vi "Bind Port.vi"(6 "timeout ms":i32=1000, 8 "error in":errorcluster, 10 "port":u16, 11 "NetStream in":refnum<class "NetStream.lvclass">) -> (0 "error out":errorcluster, 2 "Remote connected?":bool, 3 "NetStream out":refnum<class "NetStream.lvclass">)   [LabVIEW 2014, in "hse-network.lvlib" / "NetStream.lvclass"]
uses:
  NetStream.lvclass
  NetStream.lvclass/NetStream.ctl
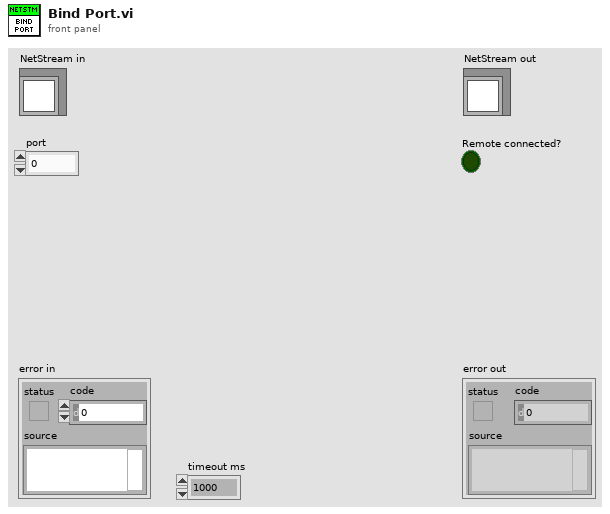
[diagram p1: front panel]
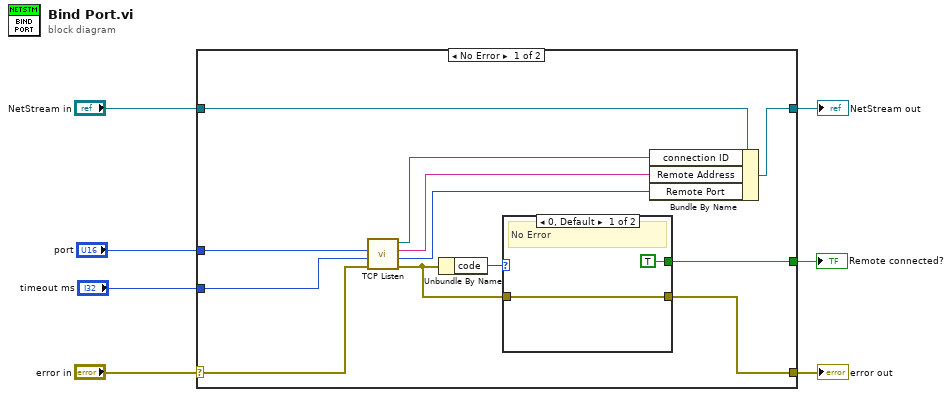
[diagram p0: block diagram]
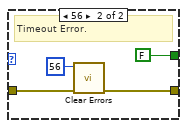
[diagram p2: hidden frame]
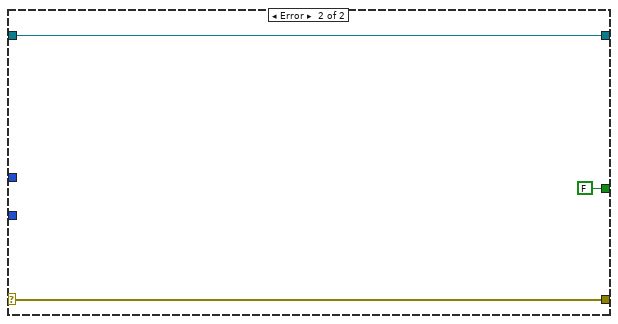
[diagram p3: hidden frame]
diagram:
  n1 = case shown="No Error" "error in" {
    selector: "error in" -> [w19 w28]
    tunnel: [w11 w28] -> w6
    tunnel: [w17 w27] -> w4
    tunnel: "NetStream in" -> [w16 w27]
    tunnel: "port" -> [w18 _]
    tunnel: "timeout ms" -> [w14 _]
    tunnel: [w10 FALSE] -> w1
    frame No Error {
      n2 = call <vilib>:"TCP Listen.vi"("error in (no error)"=w19, "timeout ms (wait forever: -1)"=w14, "port"=w18) -> ("error out"=w12:errorcluster, "remote port"=w8:u16, "remote address"=w9:string, "connection ID"=w15:refnum<k5>)  [unwired: 4 in, 1 out]
      n3 = Unbundle By Name(w12) -> ("code"=w13:i32)
      n4 = case shown="0, Default" w13 {
        tunnel: w12 -> [w21 w25]
        tunnel: [w21 w23] -> w11
        tunnel: [TRUE FALSE] -> w10
        frame 0, Default {
          # "No Error"
        }
        frame 56 {
          # "Timeout Error."
          n5 = call <vilib>:"Clear Errors.vi"("error in (no error)"=w25, "specific error code to clear (0: all)"=56) -> ("error out"=w23:errorcluster)  [unwired: 4 in, 1 out]
        }
      }
      n6 = Bundle By Name(cluster=w16, "connection ID"=w15, "Remote Address"=w9, "Remote Port"=w8) -> (w17:refnum<class "NetStream.lvclass">)
    }
    frame Error {
    }
  }
  "error out" <- w6
  "NetStream out" <- w4
  "Remote connected?" <- w1
